vi "M08 Hydro pool.vi"(11 "EV3 in":T1) -> ()   [LabVIEW 2016]
uses:
  <vilib>/NXT/Subs/LVHSConnector.ctl
  <vilib>/NXT/LegoClasses/BrickReference/BrickReference.lvclass
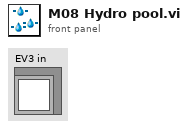
[diagram p1: front panel]
types:
  T1 = typedef "LVHSConnector.ctl" = refnum<class "BrickReference.lvclass">
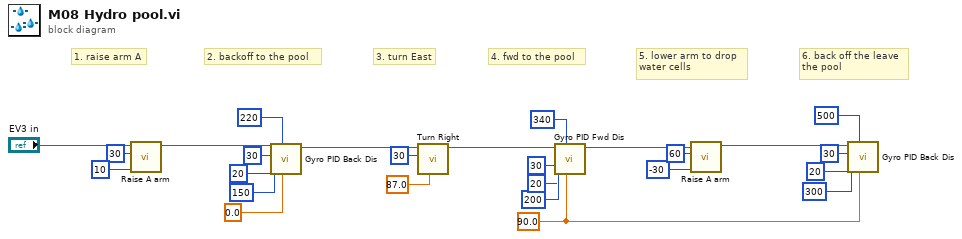
[diagram p0: block diagram]
diagram:
  w1 = sgl 90.0 ("Target angle")
  # "6. back off the leave\nthe pool"
  # "5. lower arm to drop\nwater cells"
  # "4. fwd to the pool"
  # "3. turn East"
  # "2. backoff to the pool"
  # "1. raise arm A"
  n1 = call "Raise A arm.vi"("Power"=i8 10, "Rotation"=30, "EV3 in"="EV3 in") -> ("EV3 out"=w24:T1)  [unwired: 8 in]
  n2 = call "Gyro PID Back Dis.vi"("Target angle"=sgl 0.0, "Threshold to stop"=220, "Threshold to slow"=150, "Min. speed"=20, "Max. speed"=30, "EV3 in"=w24) -> ("EV3 out"=w16:T1)  [unwired: 5 in]
  n3 = call "Turn Right.vi"("Turning angle"=sgl 87.0, "Motor B (right)"=i8 30, "EV3 in"=w16) -> ("EV3 out"=w11:T1)  [unwired: 8 in]
  n4 = call "Gyro PID Fwd Dis.vi"("Target angle"=w1, "Threshold to stop"=340, "Threshold to slow"=200, "Min. speed"=20, "Max. speed"=30, "EV3 in"=w11) -> ("EV3 out"=w8:T1)  [unwired: 5 in]
  n5 = call "Raise A arm.vi"("Power"=i8 -30, "Rotation"=60, "EV3 in"=w8) -> ("EV3 out"=w4:T1)  [unwired: 8 in]
  n6 = call "Gyro PID Back Dis.vi"("Target angle"=w1, "Threshold to stop"=500, "Threshold to slow"=300, "Min. speed"=20, "Max. speed"=30, "EV3 in"=w4) -> ()  [unwired: 5 in, 1 out]
